vi "Get Channel Data.vi"(8 "error in":errorcluster, 11 "Channel Ref in":refnum<data-value>) -> (0 "error out":errorcluster, 2 "Channel Data":T1, 3 "Channel Ref out":refnum<data-value>)   [LabVIEW 2024, in "Config File Parser.lvlib" / "Channel.lvclass"]
uses:
  Channel.lvclass
  Channel.lvclass/Channel.ctl
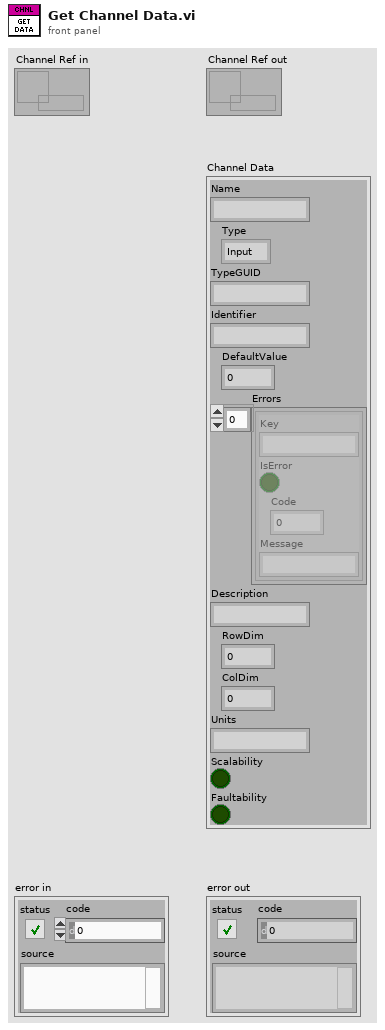
[diagram p1: front panel]
types:
  T1 = cluster{"Name":string, "Type":enum16{"Input", "Output"}, "TypeGUID":string, "Identifier":string, "DefaultValue":dbl, "Errors":cluster{"Key":string, "IsError":bool, "Code":u32, "Message":string}[], "Description":string, "RowDim":i32, "ColDim":i32, "Units":string, "Scalability":bool, "Faultability":bool}
  T2 = cluster{"Key":string, "IsError":bool, "Code":u32, "Message":string}[]
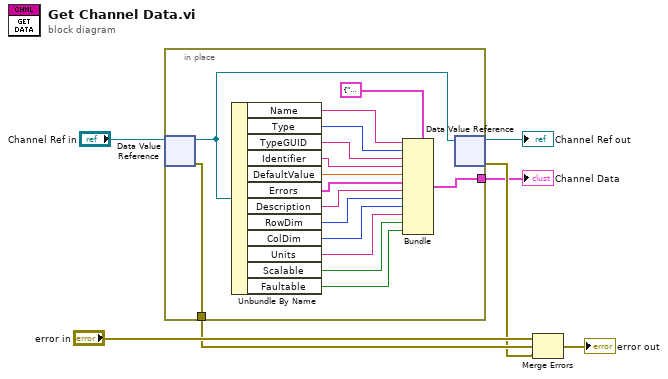
[diagram p0: block diagram]
diagram:
  n1 = in-place "In Place Element Structure" {
    in-place-border: [w22] -> w1
    in-place-border: [w23] -> w6
    n2 = in-place-dvr #1("Channel Ref in") -> (w21:refnum<class "Channel.lvclass">, w23:errorcluster)
    n3 = Unbundle By Name(w21) -> ("Name"=w20:string, "Type"=w19:enum16{"Input", "Output"}, "TypeGUID"=w18:string, "Identifier"=w17:string, "DefaultValue"=w16:dbl, "Errors"=w15:T2, "Description"=w14:string, "RowDim"=w13:i32, "ColDim"=w12:i32, "Units"=w11:string, "Scalable"=w10:bool, "Faultable"=w9:bool)
    n4 = Bundle(cluster=T1 {"Name"="", "Type"=enum."Input", "TypeGUID"="", "Identifier"="", "DefaultValue"=0.0, "Errors"=[], "Description"="", "RowDim"=0, "ColDim"=0, "Units"="", "Scalability"=FALSE, "Faultability"=FALSE}, "Name"=w20, "Type"=w19, "TypeGUID"=w18, "Identifier"=w17, "DefaultValue"=w16, "Errors"=w15, "Description"=w14, "RowDim"=w13, "ColDim"=w12, "Units"=w11, "Scalability"=w10, "Faultability"=w9) -> (w22:T1)
    n5 = in-place-dvr #1(w21) -> (→"Channel Ref out":refnum<data-value>, w5:errorcluster)
  }
  "Channel Data" <- w1
  n6 = Merge Errors("error in", w6, w5) -> (→"error out":errorcluster)
